vi "Multilabel_Confusion_Matrix.vi"(6 "Type y_pred":T1(ring), 7 "Type y_true":T1(ring), 8 "error in (no error)":errorcluster caption="entrée d'erreur (pas d'erreur)", 9 "y_pred":string[][](array[string]), 10 "y_true":string[][](array[string]), 11 "multilabel_confusion_matrix":T3={"sample_weight"=[], "labels"={"dtype_labels"="None", "labels"=["None"]}, "samplewise"=FALSE}) -> (0 "error out":errorcluster caption="sortie d'erreur", 3 "Data":T2)   [LabVIEW 2020]
doc: "Compute a confusion matrix for each class or sample\n\nCompute class-wise (default) or sample-wise (samplewise=True) multilabel confusion matrix to evaluate the accuracy of a classification, and output confusion matrices for each class or sample.\n\nIn multilabel confusion matrix MCM , the count of true negatives is MCM(0,0) , false negatives is MCM(1,0), true positives is MCM(1,1) and false positives is MCM(0,1).\n\nMulticlass data will be treated as if binarized under a one-vs-rest transformation. Returned confusion matrices will be in the order of sorted unique labels in the union of (y_true, y_pred).\n\n\nParameters : \n\n- y_true : 1d array-like, or label indicator array / sparse matrix\nof shape (n_samples, n_outputs) or (n_samples,) Ground truth (correct) target values.\n\n- y_pred : 1d array-like, or label indicator array / sparse matrix\nof shape (n_samples, n_outputs) or (n_samples,) Estimated targets as returned by a classifier\n\n- sample_weight : array-like of shape (n_samples,), default=None\nSample weights\n\n- labels : array-like\nA list of classes or column indices to select some (or to force inclusion of classes absent from the data)\n\n- samplewise : bool, default=False\nIn the multilabel case, this calculates a confusion matrix per sample\n\nReturns : \n\n- multi_confusion : array, shape (n_outputs, 2, 2)\nA 2x2 confusion matrix corresponding to each output in the input. When calculating class-wise multi_confusion (default), then n_outputs = n_labels; when calculating sample-wise multi_confusion (samplewise=True), n_outputs = n_samples. If labels is defined, the results will be returned in the order specified in labels, otherwise the results will be returned in sorted order by default."
uses:
  Multilabel_Confusion_Matrix.lvclass
panel:
  out "Multilabel_Confusion_Matrix.lvclass":refnum<class "Multilabel_Confusion_Matrix.lvclass">
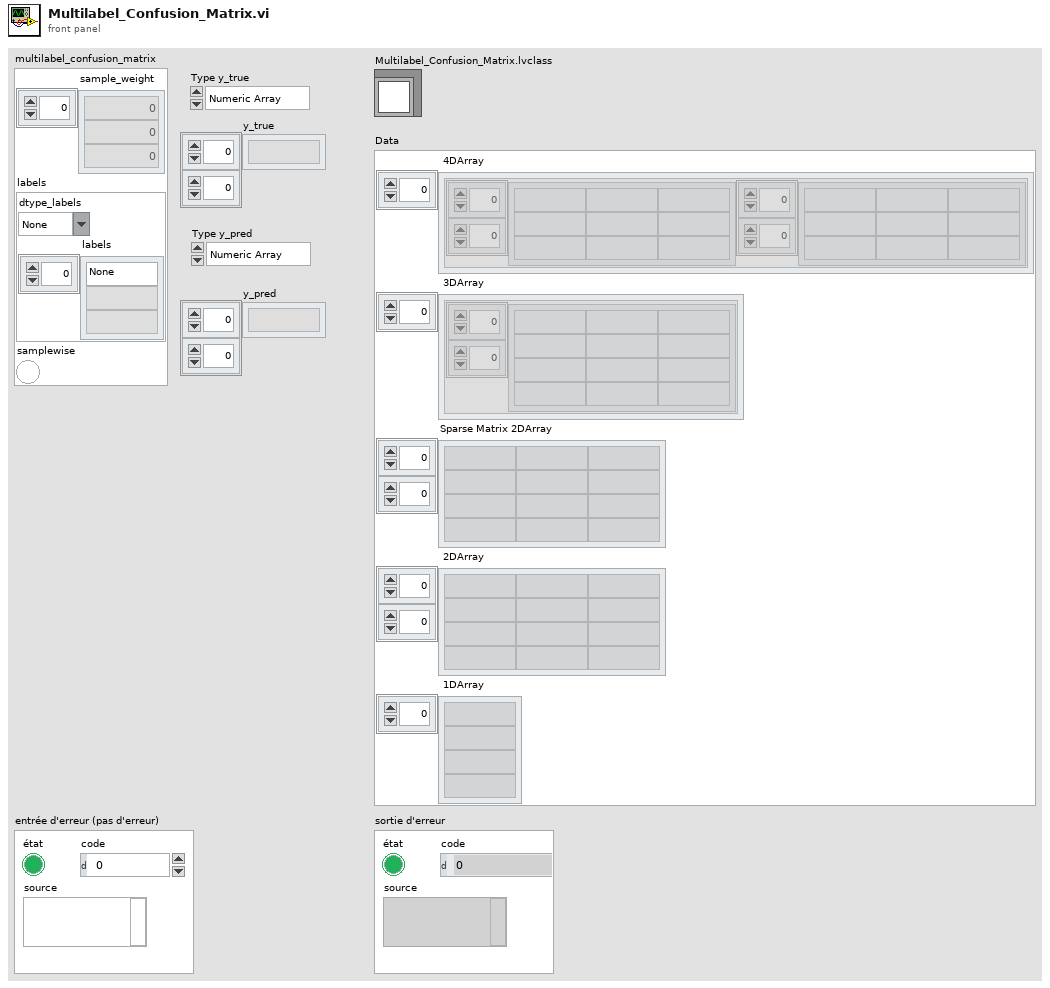
[diagram p1: front panel]
types:
  T1 = enum16{"Numeric Array", "String Array", "Sparse"}
  T2 = cluster{" 4DArray":cluster{"1":string[][], "2":string[][]}[], " 3DArray":cluster{"Tableau":string[][]}[], "Sparse Matrix 2DArray":string[][], " 2DArray":string[][], " 1DArray":string[]}
  T3 = cluster{"sample_weight":dbl[], "labels":cluster{"dtype_labels":string, "labels":string[]}, "samplewise":bool}
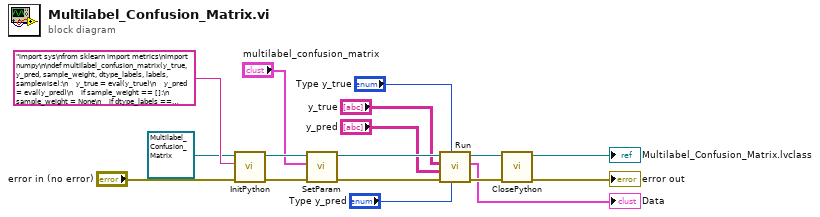
[diagram p0: block diagram]
diagram:
  n1 = call-dynamic "InitPython.vi"("error in (no error)"="error in (no error)", "Python Instruction"="import sys\nfrom sklearn import metrics\nimport numpy\n\ndef multilabel_confusion_matrix(y_true, y_pred, sample_weight, dtype_labels, labels, samplewise):\n    y_true = eval(y_true)\n    y_pred = eval(y_pred)\n    if sample_weight == []:\n        sample_weight = None\n    if dtype_labels == 'None':\n        labels = None\n    elif dtype_labels == int:\n        labels = exec(labels)\n    else:\n        pass\n    try:\n        multilabel_confusion_matrix = metrics.multilabel_confusion_matrix(y_true, y_pred, sample_weight, labels, samplewise)\n        multilabel_confusion_matrix = multilabel_confusion_matrix.tolist()\n        return str(multilabel_confusion_matrix)\n    except:\n        erreur = sys.exc_info()\n        typerr = u\"%s\" % (erreur[0])\n        typerr = typerr[typerr.find(\"'\")+1:typerr.rfind(\"'\")]\n        msgerr = u\"%s\" % (erreur[1])\n        message = str('/!\\\\ {0} : {1}'. format(typerr,msgerr))\n        return message", "Scikit-learn en entrée"=refnum<class "Multilabel_Confusion_Matrix.lvclass"> refnum ("Multilabel_Confusion_Matrix.lvclass")) -> ("error out"=w14:errorcluster, "Scikit-learn en sortie"=w13:refnum<class "Multilabel_Confusion_Matrix.lvclass">)  [unwired: 7 in]
  n2 = call-dynamic "SetParam.vi"("error in (no error)"=w14, "multilabel_confusion_matrix"="multilabel_confusion_matrix", "Multilabel_Confusion_Matrix.lvclass"=w13) -> ("error out"=w11:errorcluster, "Multilabel_Confusion_Matrix.lvclass"=w10:refnum<class "Multilabel_Confusion_Matrix.lvclass">)  [unwired: 7 in]
  n3 = call-dynamic "Run.vi"("Type y_pred"="Type y_pred", "Type y_true"="Type y_true", "error in (no error)"=w11, "y_pred"="y_pred", "y_true"="y_true", "Multilabel_Confusion_Matrix.lvclass"=w10) -> ("error out"=w9:errorcluster, "Data"=→"Data":T2, "Multilabel_Confusion_Matrix.lvclass"=w8:refnum<class "Multilabel_Confusion_Matrix.lvclass">)  [unwired: 3 in]
  n4 = call-dynamic "ClosePython.vi"("error in (no error)"=w9, "Scikit-learn en entrée"=w8) -> ("error out"=→"error out":errorcluster, "Scikit-learn en sortie"=→"Multilabel_Confusion_Matrix.lvclass":refnum<class "Multilabel_Confusion_Matrix.lvclass">)  [unwired: 8 in]
